vi "Seitenwechsel sperren.vi"(6 "Aktion":T1, 8 "error in (no error)":errorcluster caption="Fehler (Eingang, kein Fehler)") -> (0 "error out":errorcluster caption="Fehler (Ausgang)", 3 "für Seitenwechsel gesperrt":bool)   [LabVIEW 2020, in "EPA 1065.lvlib" / "ARN Test 1065-305.lvlib"]
uses:
  ARN Test 1065-305.lvlib
  Aktion FGV Seite sperren.ctl
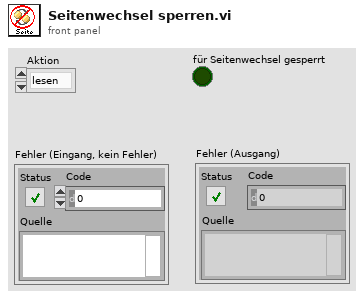
[diagram p1: front panel]
types:
  T1 = typedef "EPA 1065.lvlib/ARN Test 1065-305.lvlib/Aktion FGV Seite sperren.ctl" = enum16{"lesen", "sperren", "freigeben"}
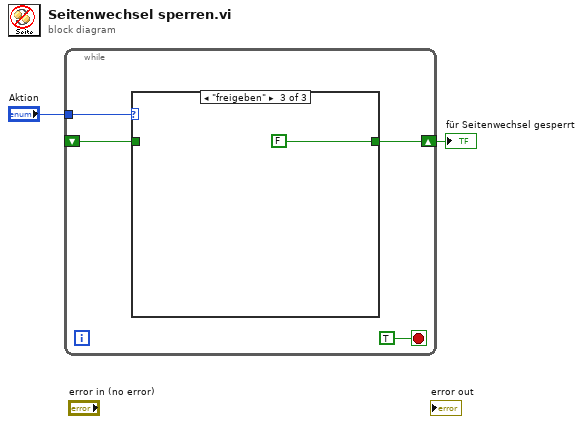
[diagram p0: block diagram]
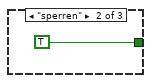
[diagram p3: hidden frame]
diagram:
  n1 = while {
    tunnel: "Aktion" -> [w5]
    shift-right: [w4] -> w1
    shift-left: _ -> [w3]
    stop <- TRUE stop-if-true
    n2 = case shown="\"freigeben\"" w5 {
      tunnel: [w7 TRUE FALSE] -> w4
      tunnel: w3 -> [w7 _ _]
      frame "lesen", Default {
      }
      frame "sperren" {
      }
      frame "freigeben" {
      }
    }
  }
  "für Seitenwechsel gesperrt" <- w1
